vi "test Compare Ports.vi"(8 "error in":errorcluster, 11 "TestCase in":refnum<class "Refresh.lvclass">) -> (0 "error out":errorcluster, 3 "TestCase out":refnum<class "Refresh.lvclass">)   [LabVIEW 2020, in "Refresh.lvclass"]
uses:
  Refresh.lvclass
  Shared/VS Channels Definition for All Labels on Hardware Channel.ctl
  Shared/VS Channels Definition for Label.ctl
  Shared/VS Channel Definition for Parameter.ctl
  Shared/Direction.ctl
  Shared/Parameter Definition.ctl
  Encoding and Decoding/Encoding.ctl
  Shared/Transfer Type.ctl
  System Explorer/Implementation/System Explorer/Types/Refresh Listbox.ctl
  System Explorer/Implementation/System Explorer/Types/Refresh Symbols.ctl
  <vilib>/addons/_JKI Toolkits/VI Tester/TestCase.llb/TestCase.lvclass
  Encoding and Decoding/Encoding and Decoding.lvlib
  System Explorer/Implementation/Implementation.lvlib
  C:/Program Files (x86)/National Instruments/LabVIEW 2020/vi.lib/addons/_JKI Toolkits/VI Tester/TestCase.llb/TestCase.lvclass
  C:/dev/niveristand-ballard-arinc429-custom-device/Source/Custom Device Support/Tests/Unit/Refresh/Refresh.lvclass
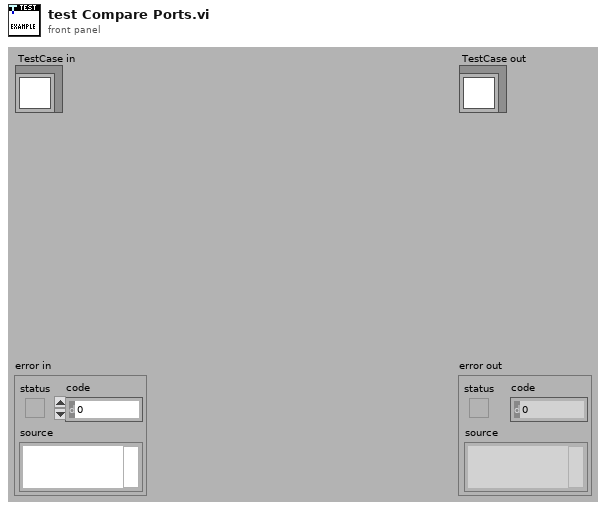
[diagram p1: front panel]
types:
  T1 = typedef "Ballard ARINC 429 System Explorer.lvlib/Implementation.lvlib/Refresh Listbox.ctl" = cluster{"Item Names":string[], "Item Symbol":T2, "Change Flag":bool}
  T2 = typedef "Ballard ARINC 429 System Explorer.lvlib/Implementation.lvlib/Refresh Symbols.ctl" = enum16{"Blank", "Port", "Incoming", "Outgoing", "Label", "Word", "Parameter", "ARINC-429", "Config Files", "Channel Spec", "Item"}
  T3 = typedef "VS Channels Definition for All Labels on Hardware Channel.ctl" = cluster{"hardware channel":i32, "labels":T4[]}
  T4 = typedef "VS Channels Definition for Label.ctl" = cluster{"label (Dec)":u32, "parameters":T5[], "SDI value":u8, "SDI enabled":bool, "transfer type":T9}
  T5 = typedef "VS Channel Definition for Parameter.ctl" = cluster{"name":string, "direction":T6, "default value":dbl, "unit":string, "Parameter":T7}
  T6 = typedef "Direction.ctl" = enum16{"Rx", "Tx"}
  T7 = typedef "Parameter Definition.ctl" = cluster{"start index":i32, "size":i32, "encoding":T8, "signed":bool, "scale multiplier":dbl, "scale offset":dbl}
  T8 = typedef "Encoding and Decoding.lvlib/Encoding.ctl" = enum16{"BNR", "BCD", "Discrete"}
  T9 = typedef "Transfer Type.ctl" = enum16{"Scheduled", "Acyclic", "Block", "Strobe"}
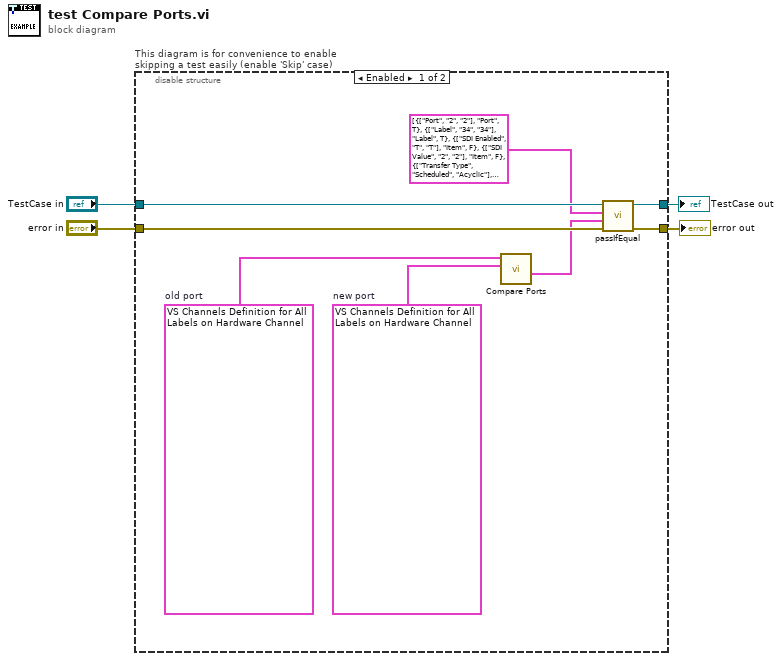
[diagram p0: block diagram]
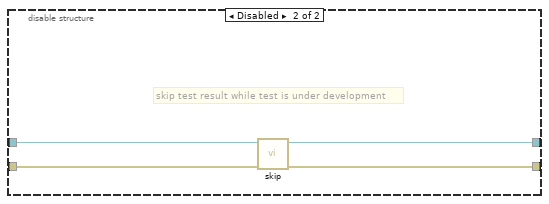
[diagram p2: hidden frame]
diagram:
  n1 = disable-structure "This diagram is for convenience to enable skipping a test easily (enable 'Skip' case)" shown="Enabled" {
    disable-tunnel: "TestCase in" -> [w12 w13]
    disable-tunnel: [w9 w14] -> w1
    disable-tunnel: [w10 w16] -> w3
    disable-tunnel: "error in" -> [w11 w15]
    frame Enabled {
      w6 = T3 {"hardware channel"=2, "labels"=[{"label (Dec)"=34, "parameters"=[{"name"="Same Name", "direction"=enum."Rx", "default value"=1.0, "unit"="psi", "Parameter"={"start index"=0, "size"=1, "encoding"=enum."BNR", "signed"=FALSE, "scale multiplier"=1.0, "scale offset"=0.0}}], "SDI value"=2, "SDI enabled"=FALSE, "transfer type"=enum."Scheduled"}]}  # old port
      w7 = T3 {"hardware channel"=2, "labels"=[{"label (Dec)"=34, "parameters"=[{"name"="Same Name", "direction"=enum."Rx", "default value"=1.0, "unit"="psi", "Parameter"={"start index"=0, "size"=1, "encoding"=enum."BNR", "signed"=FALSE, "scale multiplier"=1.0, "scale offset"=0.0}}], "SDI value"=2, "SDI enabled"=TRUE, "transfer type"=enum."Acyclic"}, {"label (Dec)"=36, "parameters"=[{"name"="New Name", "direction"=enum."Rx", "default value"=1.0, "unit"="Pa", "Parameter"={"start index"=0, "size"=1, "encoding"=enum."BNR", "signed"=FALSE, "scale multiplier"=1.0, "scale offset"=0.0}}], "SDI value"=1, "SDI enabled"=TRUE, "transfer type"=enum."Scheduled"}]}  # new port
      n2 = call "Compare Ports.vi"("new port"=w7, "old port"=w6) -> ("refresh listbox out"=w8:T1[])  [unwired: 9 in]
      n3 = call-dynamic "passIfEqual.vi"("error in (no error)"=w11, "y"=w8, "x"=T1[] [{"Item Names"=["Port", "2", "2"], "Item Symbol"=enum."Port", "Change Flag"=TRUE}, {"Item Names"=["Label", "34", "34"], "Item Symbol"=enum."Label", "Change Flag"=TRUE}, {"Item Names"=["SDI Enabled", "TRUE", "TRUE"], "Item Symbol"=enum."Item", "Change Flag"=FALSE}, {"Item Names"=["SDI Value", "2", "2"], "Item Symbol"=enum."Item", "Change Flag"=FALSE}, {"Item Names"=["Transfer Type", "Scheduled", "Acyclic"], "Item Symbol"=enum."Item", "Change Flag"=TRUE}, {"Item Names"=["Word", "", ""], "Item Symbol"=enum."Word", "Change Flag"=FALSE}, {"Item Names"=["Parameter", "Same Name", "Same Name"], "Item Symbol"=enum."Parameter", "Change Flag"=FALSE}, {"Item Names"=["Encoding", "BNR", "BNR"], "Item Symbol"=enum."Item", "Change Flag"=FALSE}, {"Item Names"=["Default Value", "1.000000", "1.000000"], "Item Symbol"=enum."Item", "Change Flag"=FALSE}, {"Item Names"=["Start Index", "0", "0"], "Item Symbol"=enum."Item", "Change Flag"=FALSE}, {"Item Names"=["Size", "1", "1"], "Item Symbol"=enum."Item", "Change Flag"=FALSE}, {"Item Names"=["Signed", "FALSE", "FALSE"], "Item Symbol"=enum."Item", "Change Flag"=FALSE}, {"Item Names"=["Scale Factor", "1.000000", "1.000000"], "Item Symbol"=enum."Item", "Change Flag"=FALSE}, {"Item Names"=["Scale Offset", "0.000000", "0.000000"], "Item Symbol"=enum."Item", "Change Flag"=FALSE}, {"Item Names"=["Unit", "psi", "psi"], "Item Symbol"=enum."Item", "Change Flag"=FALSE}, {"Item Names"=["Label", "", "36"], "Item Symbol"=enum."Label", "Change Flag"=TRUE}, {"Item Names"=["SDI Enabled", "", "TRUE"], "Item Symbol"=enum."Item", "Change Flag"=TRUE}, {"Item Names"=["SDI Value", "", "1"], "Item Symbol"=enum."Item", "Change Flag"=TRUE}, {"Item Names"=["Transfer Type", "", "Scheduled"], "Item Symbol"=enum."Item", "Change Flag"=TRUE}, {"Item Names"=["Word", "", ""], "Item Symbol"=enum."Word", "Change Flag"=TRUE}, {"Item Names"=["Parameter", "", "New Name"], "Item Symbol"=enum."Parameter", "Change Flag"=TRUE}, {"Item Names"=["Encoding", "", "BNR"], "Item Symbol"=enum."Item", "Change Flag"=TRUE}, {"Item Names"=["Default Value", "", "1.000000"], "Item Symbol"=enum."Item", "Change Flag"=TRUE}, {"Item Names"=["Start Index", "", "0"], "Item Symbol"=enum."Item", "Change Flag"=TRUE}, {"Item Names"=["Size", "", "1"], "Item Symbol"=enum."Item", "Change Flag"=TRUE}, {"Item Names"=["Signed", "", "FALSE"], "Item Symbol"=enum."Item", "Change Flag"=TRUE}, {"Item Names"=["Scale Factor", "", "1.000000"], "Item Symbol"=enum."Item", "Change Flag"=TRUE}, {"Item Names"=["Scale Offset", "", "0.000000"], "Item Symbol"=enum."Item", "Change Flag"=TRUE}, {"Item Names"=["Unit", "", "Pa"], "Item Symbol"=enum."Item", "Change Flag"=TRUE}] ("refresh listbox out"), "TestCase in"=w12) -> ("error out"=w10:errorcluster, "TestCase out"=w9:refnum<class "Refresh.lvclass">)  [unwired: 6 in]
    }
    frame Disabled {
      # "skip test result while test is under development"
      n4 = call <vilib>:"skip.vi"("error in (no error)"=w15, "TestCase in"=w13) -> ("error out"=w16:errorcluster, "TestCase out"=w14:refnum<class "Refresh.lvclass">)  [unwired: 8 in]
    }
  }
  "error out" <- w3
  "TestCase out" <- w1
